vi "ArmSetRLEDemand.vi"(9 "SetExtendPositonDemand(in)":dbl, 10 "SetLIftPostionDemand(d)":dbl, 11 "SetRotatePostionDemand(d)":dbl) -> ()   [LabVIEW 2020]
doc: "Setters for Arm\nInputs:\n--SetRotatePositionDemand(d)--\n--SetLiftPostionDemand(d)--\n--SetExtendPostionDemand(in)--"
uses:
  ArmGlobal.vi
  <vilib>/Rock Robotics/WPI/ThirdParty/JAS_Junk/TrajLib/Trajectory_Library.lvlib
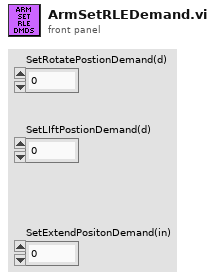
[diagram p1: front panel]
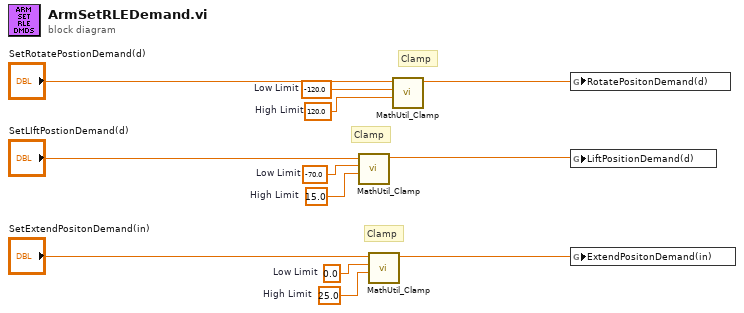
[diagram p0: block diagram]
diagram:
  w4 = 120.0  # High Limit
  w3 = -120.0  # Low Limit
  w8 = 15.0  # High Limit
  w7 = -70.0  # Low Limit
  w12 = 25.0  # High Limit
  w11 = 0.0  # Low Limit
  # "Clamp"
  # "Clamp"
  # "Clamp"
  n1 = call <vilib>:"MathUtil_Clamp.vi"("High Limit"=w8, "Low Limit"=w7, "Value"="SetLIftPostionDemand(d)") -> ("Result"=w5:dbl)  [unwired: 8 in]
  n2 = call <vilib>:"MathUtil_Clamp.vi"("High Limit"=w12, "Low Limit"=w11, "Value"="SetExtendPositonDemand(in)") -> ("Result"=w9:dbl)  [unwired: 8 in]
  n3 = call <vilib>:"MathUtil_Clamp.vi"("High Limit"=w4, "Low Limit"=w3, "Value"="SetRotatePostionDemand(d)") -> ("Result"=w1:dbl)  [unwired: 8 in]
  n4 = global write "ArmGlobal.vi" "RotatePositonDemand(d)"(w1) -> ()
  n5 = global write "ArmGlobal.vi" "LiftPositionDemand(d)"(w5) -> ()
  n6 = global write "ArmGlobal.vi" "ExtendPositonDemand(in)"(w9) -> ()
